vi "DB - [Config].[TabLabel].vi"(4 "[LanguageId]":string="en", 5 "Application":string, 6 "[SolutionId]":string="4070", 7 "DB Connection":T2={"Open"=TRUE, "Close"=TRUE}, 8 "error in (no error)":errorcluster, 11 "connection reference":T1) -> (0 "SUMMARY":errorcluster, 1 "1D data":string[](array[string]), 3 "connection reference":T1)   [LabVIEW 2013]
doc: "-- Reinehold Systems Solutions\n--\n-- 2015-01-12 21:22\n--\n\nUSE [<DB>]\nSELECT \n [Tab0Label], [Tab1Label], [Tab2Label], [Tab3Label], [Tab4Label]\n ,[Tab5Label], [Tab6Label], [Tab7Label], [Tab8Label], [Tab9Label]\n ,[Tab10Label] ,[Tab11Label] ,[Tab12Label] ,[Tab13Label] ,[Tab14Label]\n ,[Tab15Label] ,[Tab16Label] ,[Tab17Label] ,[Tab18Label] ,[Tab19Label]\n \n FROM [Config].[TabLabel] \n\nWHERE [SolutionId] = 'CMS' AND [Inactive] = '0' AND [LanguageId] = 'en' \n\nWHERE a.[PlantId] = '4070' AND a.[Inactive] = '0' AND b.[Inactive] = '0'"
uses:
  <vilib>/addons/database/Connection.llb/Conn ObjectReference.ctl
  Controls/DB - OpenClose.ctl
  Controls/Global SRTRS.vi
  Controls/Global CMS.vi
  Controls/Global AMS.vi
  <vilib>/addons/database/Connection.llb/Conn Execute.vi
  <vilib>/addons/database/Recordset.llb/Rec Fetch Recordset Data (R).vi
  <vilib>/addons/database/Recordset.llb/Rec Destroy - Connection.vi
  <vilib>/addons/database/Connection.llb/DB Tools Open Connec (String).vi
  <vilib>/addons/database/_DB Variant To Data/Database Variant To Data.xnode
  <vilib>/addons/database/NI_Database_API.lvlib
panel:
  out "Close":errorcluster
  out "SQL Statement":string
  out "2D data (NA)":string[][](array[string])
  out "DB.Config.TabLabel":string="SRTRS.Config.Plant"
  out "Connection Information":T3={"Connection "="SQL Server 32bit HPEnvy", "Username"="admin", "Password"="admin123"}
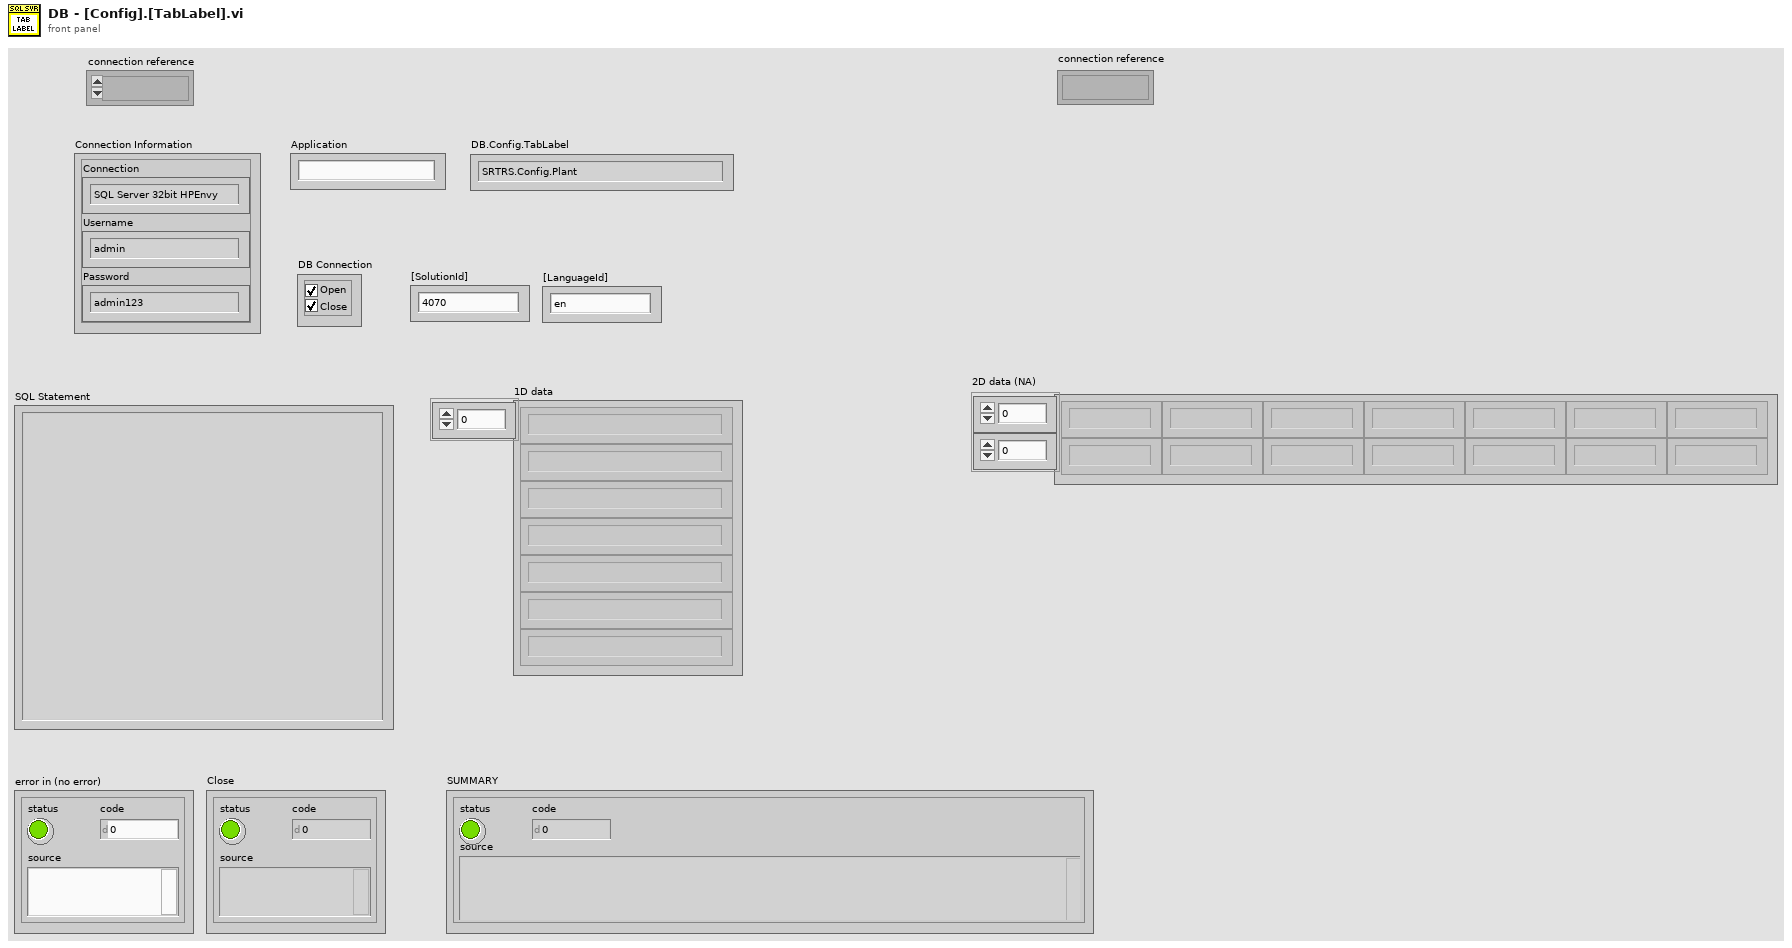
[diagram p1: front panel]
types:
  T1 = typedef "NI_Database_API.lvlib/Conn ObjectReference.ctl" = refnum<k1>
  T2 = typedef "DB - OpenClose.ctl" = cluster{"Open":bool, "Close":bool}
  T3 = cluster{"Connection ":string, "Username":string, "Password":string}
  T4 = typedef "Enum - InteractiveMode-SubVIMode.ctl" = enum16{"Interactive", "subVI Mode"}
  T5 = typedef "Connection Information Cluster.ctl" = cluster{"Connection ":string, "Username":string, "Password":string}
  T6 = typedef "DB - DB.Schema.Table.ctl" = cluster{"DB":string, "Schema":string, "Table":string}
  T7 = typedef "NI_Database_API.lvlib/Rec ObjectReference.ctl" = refnum<k1>
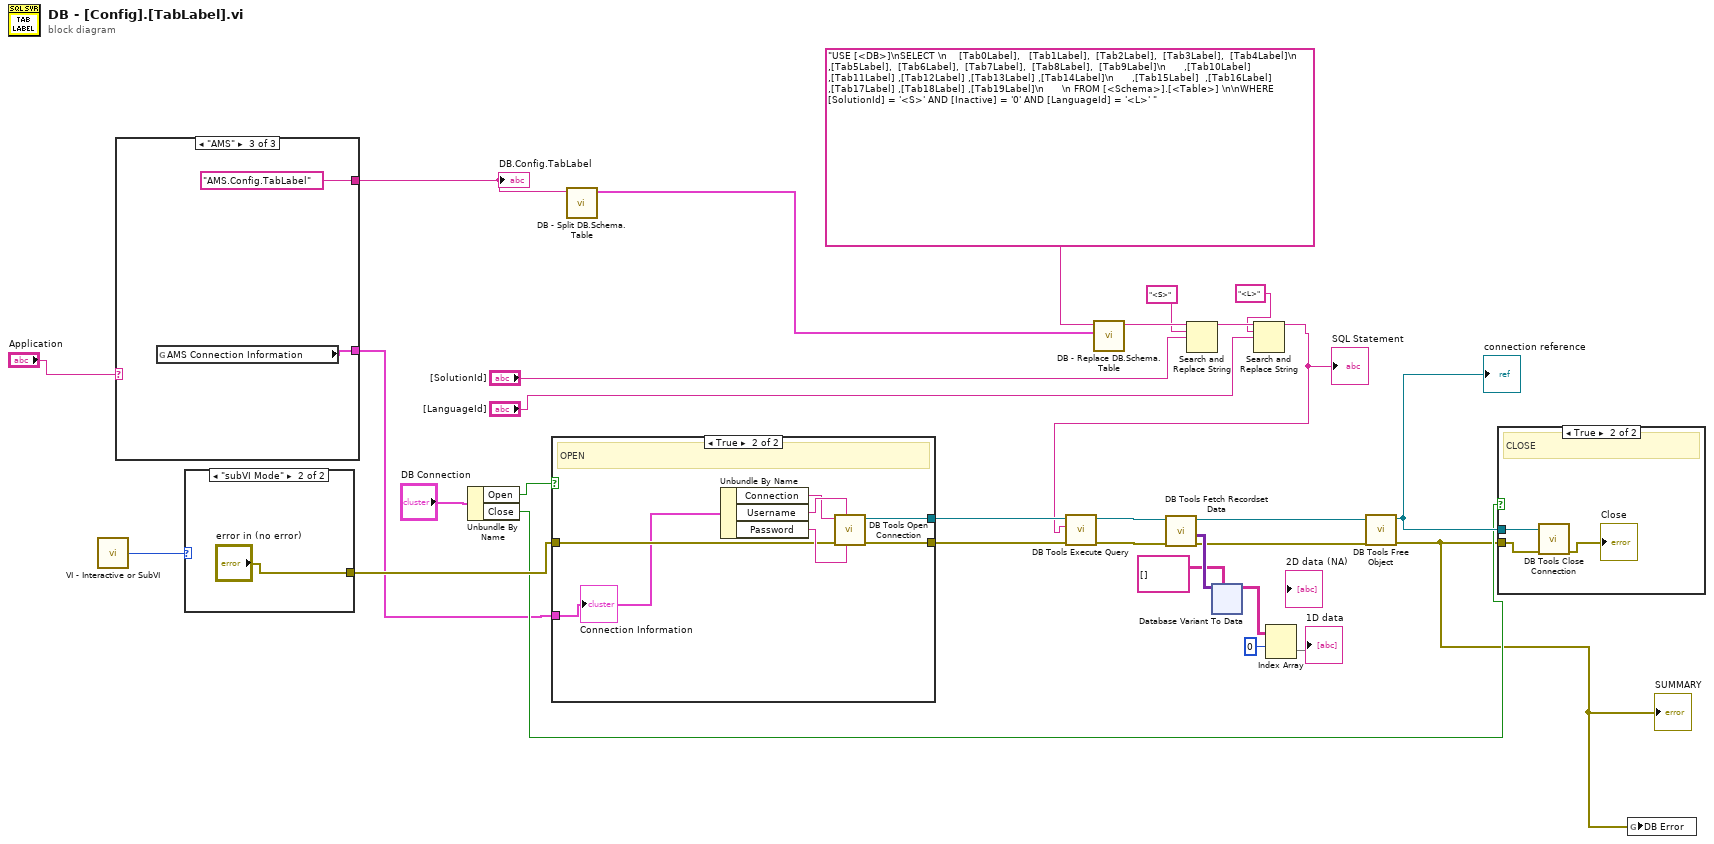
[diagram p0: block diagram]
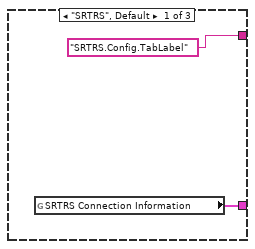
[diagram p2: hidden frame]
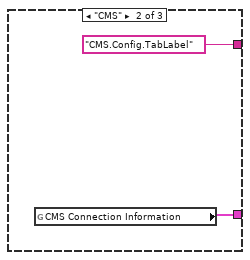
[diagram p3: hidden frame]
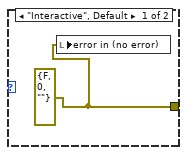
[diagram p5: hidden frame]
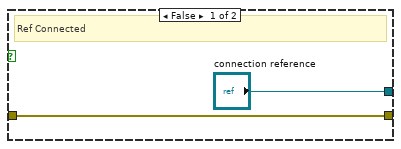
[diagram p6: hidden frame]
diagram:
  n1 = call "VI - Interactive or SubVI.vi"() -> ("Mode"=w28:T4)  [unwired: 5 in]
  n2 = case shown="\"AMS\"" "Application" {
    tunnel: [w32 w34 w35] -> w6
    tunnel: ["SRTRS.Config.TabLabel" ("DB.Schema.Table\nSRTRS.Config.Plant") "CMS.Config.TabLabel" ("DB.Schema.Table\nSRTRS.Config.Plant") "AMS.Config.TabLabel" ("DB.Schema.Table\nSRTRS.Config.Plant")] -> w5
    frame "SRTRS", Default {
      n3 = global read "Global SRTRS.vi" "SRTRS Connection Information"() -> (w32:T5)
    }
    frame "CMS" {
      n4 = global read "Global CMS.vi" "CMS Connection Information"() -> (w34:T5)
    }
    frame "AMS" {
      n5 = global read "Global AMS.vi" "AMS Connection Information"() -> (w35:T5)
    }
  }
  "DB.Config.TabLabel" <- w5
  n6 = case shown="\"subVI Mode\"" w28 {
    tunnel: [w37 "error in (no error)"] -> w27
    frame "Interactive", Default {
      w37 = errorcluster {"status"=FALSE, "code"=0, "source"=""} ("error in (no error)")
      n7 = local write "error in (no error)"(w37) -> ()
    }
    frame "subVI Mode" {
    }
  }
  n8 = Unbundle By Name("DB Connection") -> ("Open"=w29:bool, "Close"=w17:bool)
  n9 = case shown="True" w29 {
    tunnel: ["connection reference" w44] -> w20
    tunnel: w27 -> [w39 w43]
    tunnel: [w39 w42] -> w19
    tunnel: w6 -> [_ w41]
    frame False {
      # "Ref Connected"
    }
    frame True {
      # "OPEN"
      n10 = Unbundle By Name(w41) -> ("Connection"=w46:string, "Username"=w47:string, "Password"=w45:string)
      n11 = call-poly <vilib>:"DB Tools Open Connection.vi"("password"=w45, "userID"=w47, "error in (no error)"=w43, "connection information"=w46) -> ("error out"=w42:errorcluster, "connection reference"=w44:T1)  [unwired: 4 in]
      "Connection Information" <- w41
    }
  }
  n12 = call "DB - Split DB.Schema.Table.vi"("DB.Schema.Table"=w5) -> ("DB.Schema.Table"=w16:T6)  [unwired: 10 in]
  n13 = call "DB - Replace DB.Schema.Table.vi"("DB.Schema.Table"=w16, "string in"="USE [<DB>]\nSELECT \n    [Tab0Label],   [Tab1Label],  [Tab2Label],  [Tab3Label],  [Tab4Label]\n      ,[Tab5Label],  [Tab6Label],  [Tab7Label],  [Tab8Label],  [Tab9Label]\n      ,[Tab10Label] ,[Tab11Label] ,[Tab12Label] ,[Tab13Label] ,[Tab14Label]\n      ,[Tab15Label]  ,[Tab16Label] ,[Tab17Label] ,[Tab18Label] ,[Tab19Label]\n      \n FROM [<Schema>].[<Table>] \n\nWHERE [SolutionId] = '<S>' AND [Inactive] = '0' AND [LanguageId] = '<L>' ") -> ("string out"=w14:string)  [unwired: 8 in, 1 out]
  n14 = Search and Replace String(input string=w14, search string="<S>", replace string="[SolutionId]") -> (result string=w3:string)  [unwired: 5 in, 3 out]
  n15 = Search and Replace String(input string=w3, search string="<L>", replace string="[LanguageId]") -> (result string=w4:string)  [unwired: 5 in, 3 out]
  "SQL Statement" <- w4
  n16 = call-poly <vilib>:"DB Tools Execute Query.vi"("error in (no error)"=w19, "SQL query"=w4, "connection reference"=w20) -> ("error out"=w26:errorcluster, "recordset reference"=w25:T7)  [unwired: 5 in]
  n17 = call-poly <vilib>:"DB Tools Fetch Recordset Data.vi"("error in (no error)"=w26, "recordset reference"=w25) -> ("error out"=w21:errorcluster, "recordset data"=w24:variant[][], "recordset reference out"=w22:T7)  [unwired: 3 in]
  n18 = xnode "Database Variant To Data"("database variant"=w24, "type"=string[][] []) -> ("data"=w11:string[][])  [unwired: 1 in, 1 out]
  n19 = Index Array(array=w11, index (row)=0) -> (element=→"1D data":string[])  [unwired: 1 in]
  n20 = call-poly <vilib>:"DB Tools Free Object.vi"("error in (no error)"=w21, "recordset reference"=w22) -> ("error out"=w8:errorcluster, "connection reference"=w18:T1)  [unwired: 8 in]
  "SUMMARY" <- w8
  "connection reference" <- w18
  n21 = case shown="True" w17 {
    tunnel: w18 -> [_ w50]
    tunnel: w8 -> [_ w49]
    frame False {
      # "Ref Connected"
    }
    frame True {
      # "CLOSE"
      n22 = call <vilib>:"DB Tools Close Connection.vi"("error in (no error)"=w49, "connection reference"=w50) -> ("error out"=→"Close":errorcluster)  [unwired: 5 in]
    }
  }
  n23 = global write "Global SRTRS.vi" "DB Error"(w8) -> ()
